vi "servo.vi"   [LabVIEW 2016, in "Test.lvrbt"]
uses:
  Test.lvrbt
  <vilib>/NXT/Hardware/Plugins/Tetrix 180 deg Servo/Tetrix180ServoAddress.ctl
  <vilib>/NXT/NXTIO Xnodes/NXTIONodeSubVIs/TETRIX IO Move Servos.vi
  <vilib>/NXT/Dual Mode Library/Waits/Wait_Num.vi
  <vilib>/NXT/Subs/LVHSConnector.ctl
  <vilib>/NXT/NXTIO Xnodes/AddressXNode/NXTIOAddress.xnode
  <vilib>/NXT/NXTIO Xnodes/NXTIOXNode/NXTIO.xnode
  <vilib>/NXT/LegoClasses/BrickReference/BrickReference.lvclass
types:
  T1 = typedef "Tetrix180ServoAddress.ctl" = i32
  T2 = cluster{"Tetrix180Servo":T1, "Tetrix180Servo":T1, "Tetrix180Servo":T1, "Tetrix180Servo":T1, "Tetrix180Servo":T1}
  T3 = typedef "LVHSConnector.ctl" = refnum<class "BrickReference.lvclass">
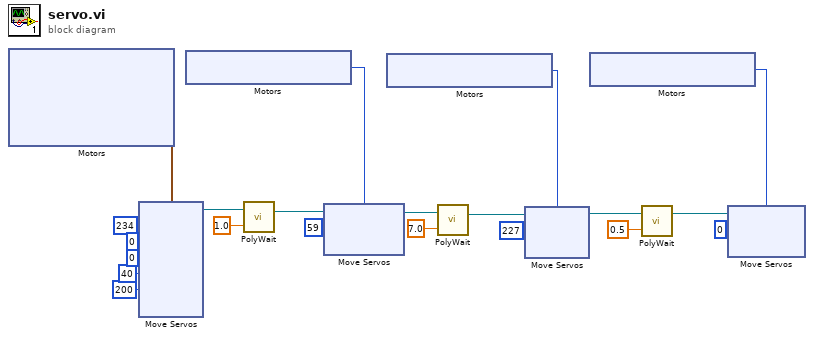
[diagram p0: block diagram]
diagram:
  n1 = xnode "Motors"() -> ("Motor"=w21:T2)
  n2 = xnode "Move Servos"("Position 5"=u8 200, "Position 4"=u8 40, "Position 3"=u8 0, "Position 2"=u8 0, "Position 1"=u8 234, "Motors"=w21) -> ("NXT/EV3"=w15:T3)  [unwired: 1 in]
  n3 = xnode "Motors"() -> ("Motor"=w12:T1)
  n4 = call-poly <vilib>:"PolyWait.vi"("Time (1 sec)"=sgl 1.0, "NXT/EV3"=w15) -> ("NXT/EV3"=w13:T3)  [unwired: 2 in]
  n5 = xnode "Move Servos"("Position 1"=u8 59, "Motors"=w12, "NXT/EV3"=w13) -> ("NXT/EV3"=w9:T3)
  n6 = xnode "Motors"() -> ("Motor"=w8:T1)
  n7 = call-poly <vilib>:"PolyWait.vi"("Time (1 sec)"=sgl 7.0, "NXT/EV3"=w9) -> ("NXT/EV3"=w6:T3)  [unwired: 2 in]
  n8 = xnode "Move Servos"("Position 1"=u8 227, "Motors"=w8, "NXT/EV3"=w6) -> ("NXT/EV3"=w4:T3)
  n9 = xnode "Motors"() -> ("Motor"=w3:T1)
  n10 = call-poly <vilib>:"PolyWait.vi"("Time (1 sec)"=sgl 0.5, "NXT/EV3"=w4) -> ("NXT/EV3"=w1:T3)  [unwired: 2 in]
  n11 = xnode "Move Servos"("Position 1"=u8 0, "Motors"=w3, "NXT/EV3"=w1) -> ()  [unwired: 1 out]
